vi "ext_trig_acquire_scmos.vi"() -> ()   [LabVIEW 2015]
panel:
  in  "Preview":bool
  in  "Frames":dbl
  out "Image":i32[][](graph)
  in  "Acquire":bool
  in  "stop button":bool caption="stop"
  out "Firmware":string
  out "Camera ID":string
  out "Model":string
  out "DCAM Ver.":string
  out "Library Ver.":string
  # "Software Information"
  # "Camera Information"
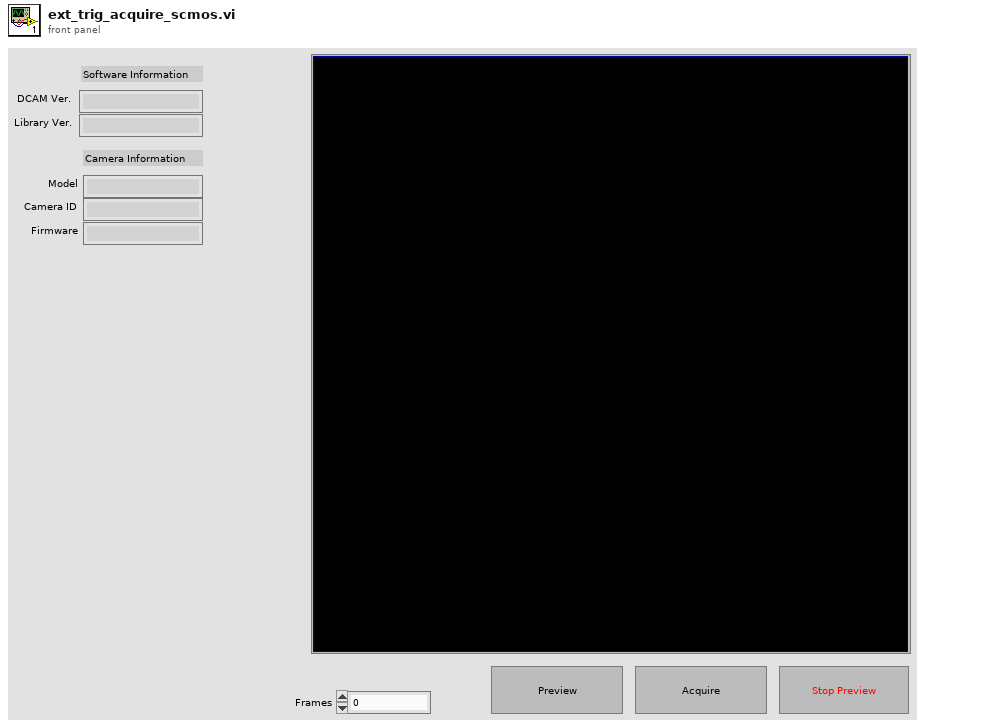
[diagram p1: front panel]
types:
  T1 = cluster{"Capture Library":string, "DCAM-API":string}
  T2 = cluster{"Mode":u32, "Polarity":u32, "Period":dbl, "Delay":dbl}
  T3 = cluster{"Mode":u32, "Polarity":u16, "Times":u32, "Delay":dbl}
  T4 = cluster{"Model":string, "Camera ID":string, "Firmware":string}
  T5 = cluster{"height":u32, "width":u32, "datatype":u32}
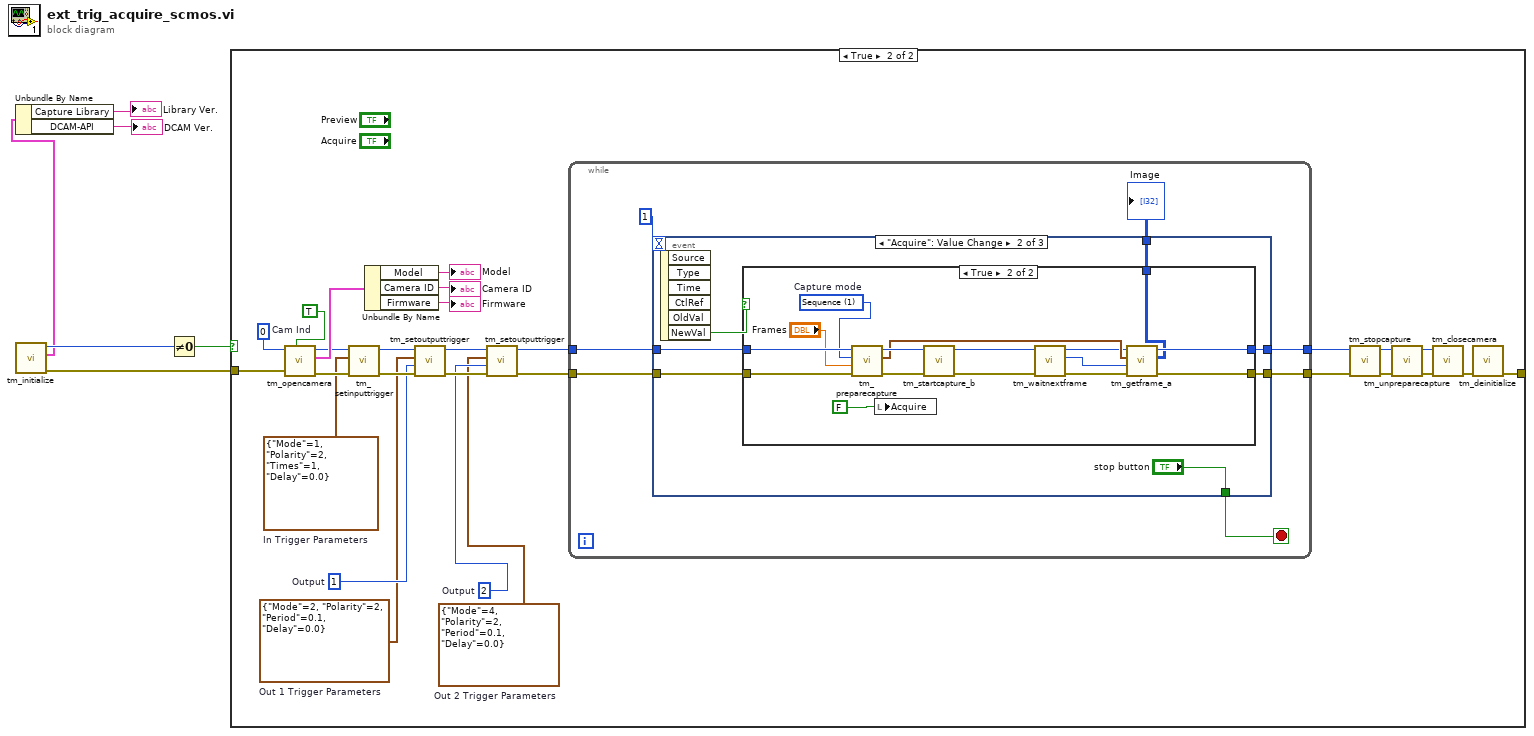
[diagram p0: block diagram]
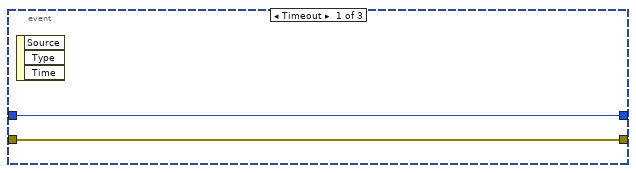
[diagram p3: hidden frame]
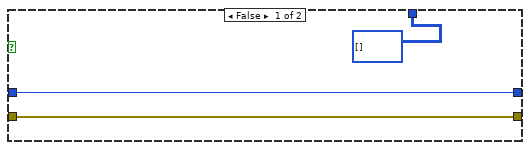
[diagram p4: hidden frame]
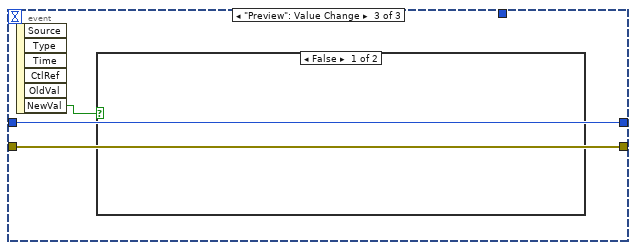
[diagram p5: hidden frame]
diagram:
  n1 = call <userlib>:"tm_initialize.vi"() -> ("error out"=w6:errorcluster, "Version Info"=w1:T1, "Number Of Cameras"=w5:u32)  [unwired: 8 in, 1 out]
  n2 = Unbundle By Name(w1) -> ("Capture Library"=→"Library Ver.":string, "DCAM-API"=→"DCAM Ver.":string)
  n3 = Not Equal To 0?(x=w5) -> (x != 0?=w4:bool)
  n4 = case shown="True" w4 {
    tunnel: w6 -> [w7 w35]
    tunnel: [w7 w33] -> _
    frame False {
    }
    frame True {
      w10 = T2 {"Mode"=4, "Polarity"=2, "Period"=0.1, "Delay"=0.0}  # Out 2 Trigger Parameters
      w11 = T2 {"Mode"=2, "Polarity"=2, "Period"=0.1, "Delay"=0.0}  # Out 1 Trigger Parameters
      w14 = 2  # Output
      w17 = 1  # Output
      w12 = T3 {"Mode"=1, "Polarity"=2, "Times"=1, "Delay"=0.0}  # In Trigger Parameters
      w34 = 0  # Cam Ind
      n5 = call <userlib>:"tm_opencamera.vi"("Force Open"=TRUE, "error in (no error)"=w35, "Camera Index"=w34) -> ("error out"=w21:errorcluster, "Camera Details"=w30:T4, "Handle out"=w20:u32)  [unwired: 6 in]
      n6 = call <userlib>:"tm_setinputtrigger.vi"("error in (no error)"=w21, "Parameters"=w12, "Handle in"=w20) -> ("error out"=w19:errorcluster, "Handle out"=w18:u32)  [unwired: 7 in]
      n7 = Unbundle By Name(w30) -> ("Model"=→"Model":string, "Camera ID"=→"Camera ID":string, "Firmware"=→"Firmware":string)
      n8 = call <userlib>:"tm_setoutputtrigger.vi"("error in (no error)"=w19, "Index"=w17, "Parameters"=w11, "Handle in"=w18) -> ("error out"=w15:errorcluster, "Handle out"=w16:u32)  [unwired: 6 in]
      n9 = call <userlib>:"tm_setoutputtrigger.vi"("error in (no error)"=w15, "Index"=w14, "Parameters"=w10, "Handle in"=w16) -> ("error out"=w9:errorcluster, "Handle out"=w8:u32)  [unwired: 6 in]
      n10 = while {
        tunnel: w9 -> [w40]
        tunnel: [w38] -> w32
        tunnel: w8 -> [w41]
        tunnel: [w42] -> w31
        stop <- w37 stop-if-true
        n11 = event shown="[1] \"Acquire\": Value Change" {
          selector: _ -> [_ _ _]
          dyn-events: _ -> [_ _ _]
          timeout: 1 -> [_ _ _]
          tunnel: [w43 w51 w73] -> w42
          tunnel: w41 -> [w43 w48 w73]
          tunnel: w40 -> [w44 w49 w72]
          tunnel: [w44 w50 w72] -> w38
          tunnel: [_ "stop button" _] -> w37
          tunnel: [_ w45 _] -> w36
          event Timeout {
            n12 = event-data() -> ()  [unwired: 1 in, 3 out]
          }
          event "Acquire": Value Change {
            n13 = event-data() -> ("NewVal"=w47:bool)  [unwired: 1 in, 5 out]
            n14 = case shown="True" w47 {
              tunnel: [w54 w70] -> w50
              tunnel: w48 -> [w53 w65]
              tunnel: w49 -> [w54 w64]
              tunnel: [w53 w69] -> w51
              tunnel: [i32[][] [] w55] -> w45
              frame False {
              }
              frame True {
                w60 = 1 items=["Snap", "Sequence"]  # Capture mode
                n15 = call <userlib>:"tm_preparecapture.vi"("error in (no error)"=w64, "Frames"="Frames", "Capture mode"=w60, "Handle in"=w65) -> ("error out"=w67:errorcluster, "Buffer Info"=w63:T5, "Handle out"=w66:u32)  [unwired: 4 in, 1 out]
                n16 = local write "Acquire"(FALSE) -> ()
                n17 = call <userlib>:"tm_startcapture_b.vi"("error in (no error)"=w67, "Handle in"=w66) -> ("error out"=w62:errorcluster, "Handle out"=w61:u32)  [unwired: 8 in]
                n18 = call <userlib>:"tm_waitnextframe.vi"("error in (no error)"=w62, "Handle in"=w61) -> ("error out"=w59:errorcluster, "Frame Index"=w57:i32, "Handle out"=w58:u32)  [unwired: 6 in, 1 out]
                n19 = call <userlib>:"tm_getframe_a.vi"("error in (no error)"=w59, "Frame Index"=w57, "Buffer Info"=w63, "Handle in"=w58) -> ("error out"=w70:errorcluster, "Data 16"=w55:u16[][], "Handle out"=w69:u32)  [unwired: 3 in, 2 out]
              }
            }
          }
          event "Preview": Value Change {
            n20 = event-data() -> ("NewVal"=w71:bool)  [unwired: 1 in, 5 out]
            n21 = case shown="False" w71 {
              frame False {
              }
              frame True {
              }
            }
          }
        }
        "Image" <- w36
      }
      n22 = call <userlib>:"tm_stopcapture.vi"("error in (no error)"=w32, "Handle in"=w31) -> ("error out"=w23:errorcluster, "Handle out"=w24:u32)  [unwired: 8 in]
      n23 = call <userlib>:"tm_unpreparecapture.vi"("error in (no error)"=w23, "Handle in"=w24) -> ("error out"=w22:errorcluster, "Handle out"=w25:u32)  [unwired: 8 in]
      n24 = call <userlib>:"tm_closecamera.vi"("error in (no error)"=w22, "Handle in"=w25) -> ("error out"=w26:errorcluster)  [unwired: 9 in]
      n25 = call <userlib>:"tm_deinitialize.vi"("error in (no error)"=w26) -> ("error out"=w33:errorcluster)  [unwired: 10 in]
    }
  }
